vi "Main.vi"() -> ()   [LabVIEW 2016]
doc: "The roboRIO Project template acquires acceleration data from the onboard accelerometer and displays the changes of acceleration values in a waveform chart."
panel:
  out "String":string
  in  "Boolean 1":bool
  in  "Boolean 2":bool
  out "Test 4":bool
  out "Finger 1 (individual) 2":bool
  out "Finger 2 (individual) 2":bool
  out "Finger 3 (individual) 2":bool
  out "Finger 4 (individual)":bool
  out "Finger 5 (individual) 2":bool
  in  "Finger 1 (individual)":bool
  in  "Finger 3 (individual)":bool
  in  "FInger 4 (individual)":bool
  in  "Finger 5 (individual)":bool
  in  "Finger 2 (individual)":bool
  in  "stop":bool
  out "Test 1":bool
  out "Test 2":bool
  out "Test 3":bool
  out "Finger 1 (thumb)":i16(knob) scale=0.0..180.0
  out "Finger 4 (ring)":i16(knob) scale=0.0..180.0
  out "Finger 3 (middle)":i16(knob) scale=0.0..180.0
  out "Finger 2 (index)":i16(knob) scale=0.0..180.0
  out "Finger 5 (little)":i16(knob) scale=0.0..180.0
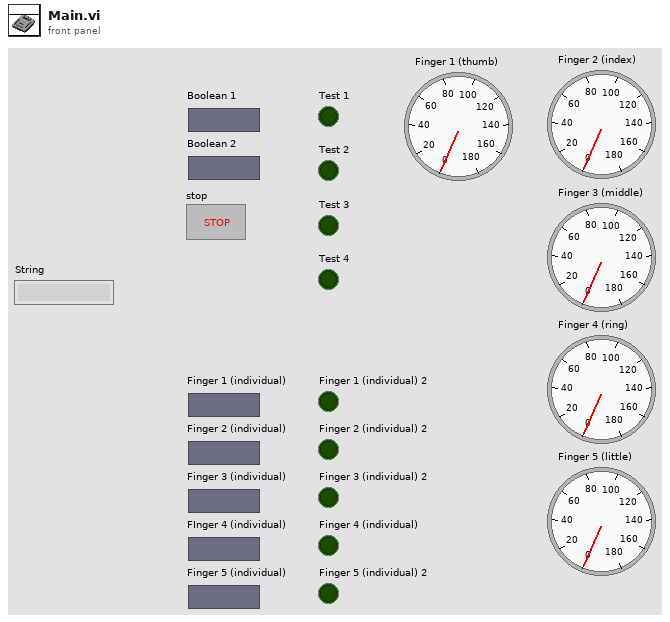
[diagram p1: front panel]
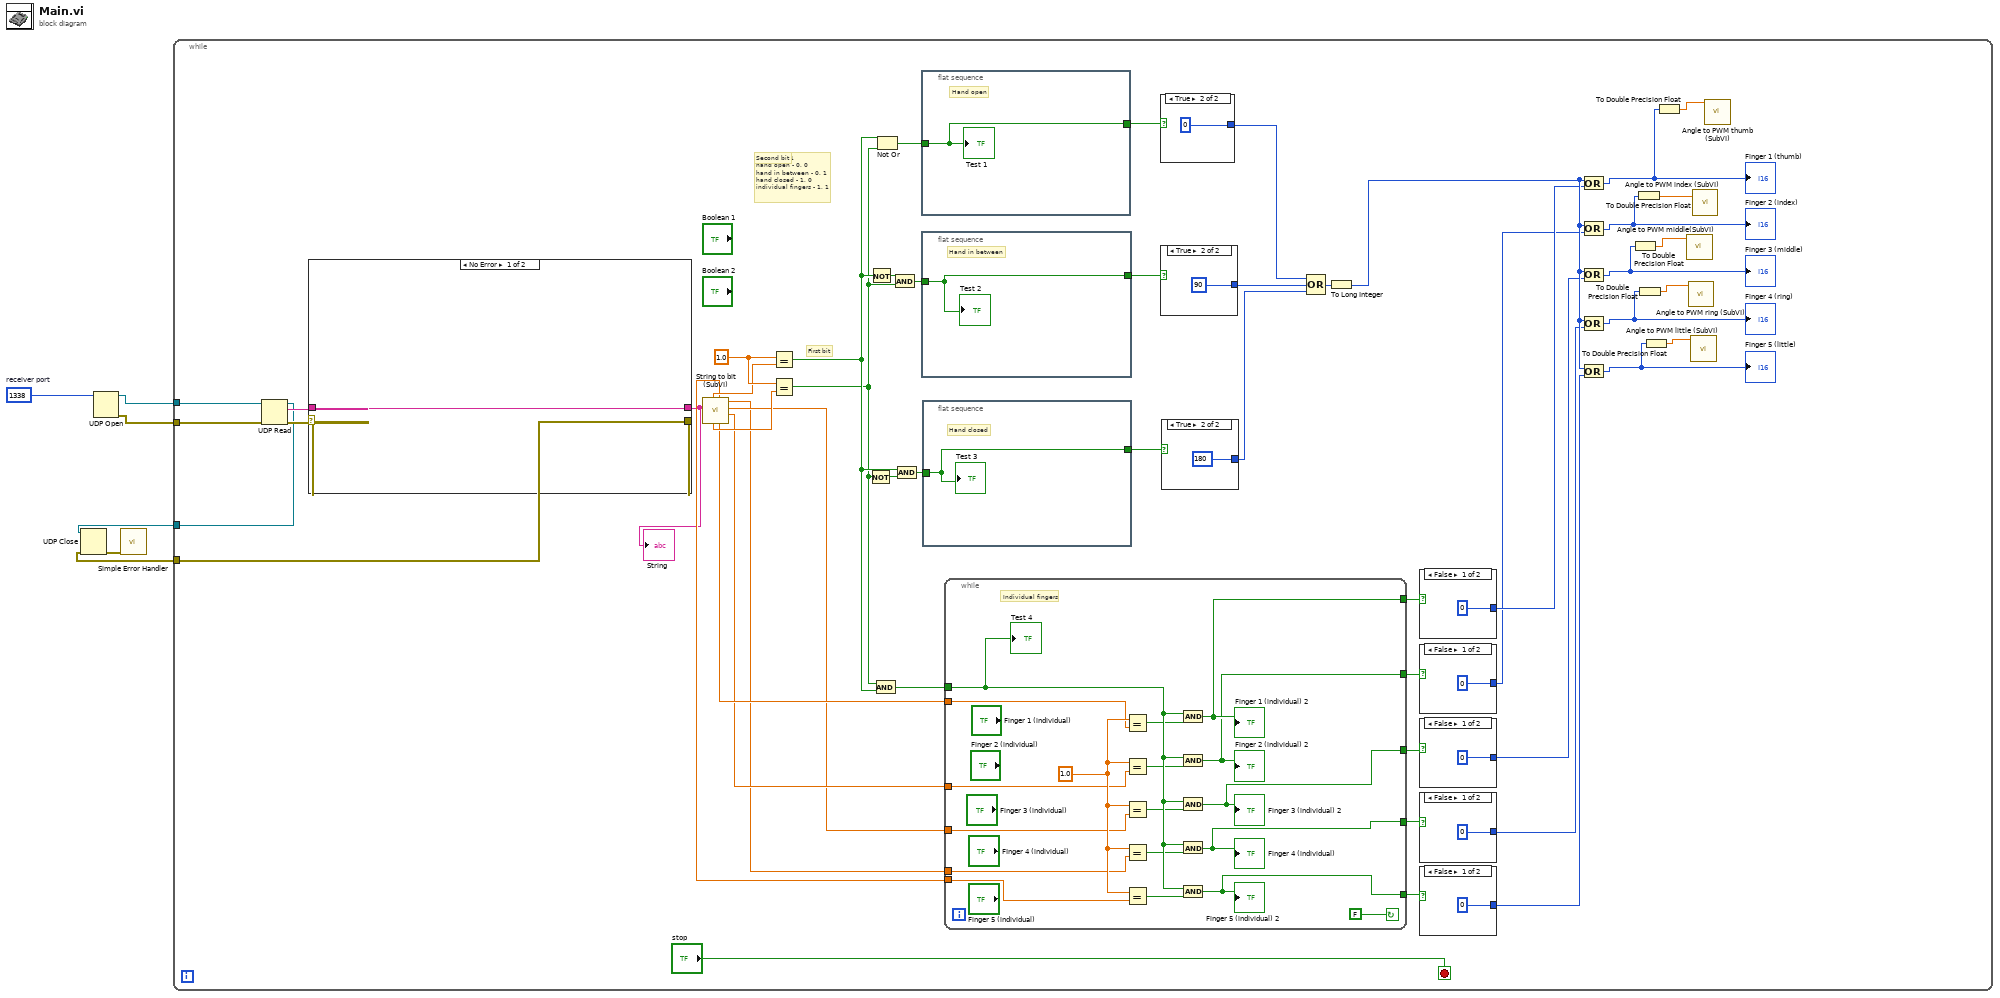
[diagram p0: block diagram]
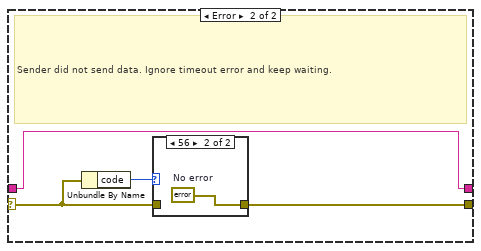
[diagram p2: hidden frame]
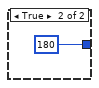
[diagram p4: hidden frame]
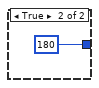
[diagram p5: hidden frame]
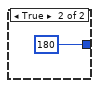
[diagram p6: hidden frame]
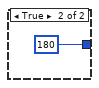
[diagram p7: hidden frame]
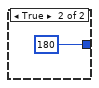
[diagram p8: hidden frame]
diagram:
  w6 = u16 1338  # receiver port
  n1 = UDP Open(11:w6) -> (port=w4:refnum<k16>, 0:w5:errorcluster)  [unwired: 4 in, 1 out]
  n2 = while {
    tunnel: w5 -> [w18]
    tunnel: w4 -> [w17]
    tunnel: [w16] -> w2
    tunnel: [w15] -> w1
    stop <- "stop" stop-if-true
    w38 = 1.0
    # "Second bit"
    # "First bit"
    # "Command 1\nhand open - 0, 0\nhand in between - 0, 1\nhand closed - 1, 0\nindividual fingers - 1, 1"
    n3 = UDP Read(connection ID=w17, 8:w18) -> (data out=w20:string, error out=w19:errorcluster, 3:w16:refnum<k16>)  [unwired: 1 in, 3 out]
    n4 = case shown="No Error" w19 {
      selector: w19 -> [w60 w63]
      tunnel: w20 -> [w59 w61]
      tunnel: [w60 w62] -> w15
      tunnel: [w59 w61] -> w7
      frame No Error {
      }
      frame Error {
        # "Sender did not send data. Ignore timeout error and keep waiting."
        n5 = Unbundle By Name(w63) -> ("code"=w64:i32)
        n6 = case shown="56" w64 {
          tunnel: w63 -> [w65 _]
          tunnel: [w65 w66] -> w62
          frame Default {
          }
          frame 56 {
            w66 = errorcluster {"status"=FALSE, "code"=0, "source"=""}  # No error
          }
        }
      }
    }
    "String" <- w7
    n7 = call "String to bit (SubVI).vi"("String in"=w7) -> ("Pointy finger"=w11:dbl, "Middle finger"=w10:dbl, "Ringfinger"=w9:dbl, "Thumb"=w12:dbl, "Lillfinger"=w8:dbl, "Command LSD"=w14:dbl, "Command MSD"=w13:dbl)  [unwired: 4 in]
    n8 = Equal?(x=w38, y=w13) -> (x = y?=w39:bool)
    n9 = Equal?(x=w38, y=w14) -> (x = y?=w37:bool)
    n10 = Not(x=w37) -> (.not. x?=w57:bool)
    n11 = Not(x=w39) -> (.not. x?=w58:bool)
    n12 = And(x=w37, y=w39) -> (x .and. y?=w56:bool)
    n13 = Not Or(1:w37, 2:w39) -> (0:w55:bool)
    n14 = And(x=w58, y=w37) -> (x .and. y?=w54:bool)
    n15 = And(x=w39, y=w57) -> (x .and. y?=w53:bool)
    n16 = flat-sequence {
      tunnel: w55 -> [w82]
      tunnel: [w82] -> w51
      frame #0 {
        # "Hand open"
        "Test 1" <- w82
      }
    }
    n17 = flat-sequence {
      tunnel: w54 -> [w81]
      tunnel: [w81] -> w52
      frame #0 {
        # "Hand in between"
        "Test 2" <- w81
      }
    }
    n18 = flat-sequence {
      tunnel: w53 -> [w80]
      tunnel: [w80] -> w49
      frame #0 {
        # "Hand closed"
        "Test 3" <- w80
      }
    }
    n19 = while {
      tunnel: w56 -> [w100]
      tunnel: [w98] -> w36
      tunnel: [w97] -> w35
      tunnel: [w96] -> w34
      tunnel: [w95] -> w33
      tunnel: [w94] -> w32
      tunnel: w12 -> [w87]
      tunnel: w11 -> [w86]
      tunnel: w10 -> [w85]
      tunnel: w9 -> [w84]
      tunnel: w8 -> [w83]
      stop <- FALSE continue-if-true
      w93 = 1.0
      # "Individual fingers"
      n20 = Equal?(x=w93, y=w87) -> (x = y?=w92:bool)
      n21 = Equal?(x=w93, y=w86) -> (x = y?=w91:bool)
      n22 = Equal?(x=w93, y=w85) -> (x = y?=w90:bool)
      n23 = Equal?(x=w93, y=w84) -> (x = y?=w89:bool)
      n24 = Equal?(x=w93, y=w83) -> (x = y?=w88:bool)
      n25 = And(x=w100, y=w92) -> (x .and. y?=w98:bool)
      "Finger 1 (individual) 2" <- w98
      n26 = And(x=w100, y=w91) -> (x .and. y?=w97:bool)
      "Finger 2 (individual) 2" <- w97
      n27 = And(x=w100, y=w90) -> (x .and. y?=w96:bool)
      "Finger 3 (individual) 2" <- w96
      n28 = And(x=w100, y=w89) -> (x .and. y?=w95:bool)
      "Finger 4 (individual)" <- w95
      n29 = And(x=w100, y=w88) -> (x .and. y?=w94:bool)
      "Finger 5 (individual) 2" <- w94
      "Test 4" <- w100
    }
    n30 = case shown="True" w51 {
      tunnel: [_ i16 0] -> w50
      frame False {
      }
      frame True {
      }
    }
    n31 = case shown="True" w52 {
      tunnel: [_ i16 90] -> w48
      frame False {
      }
      frame True {
      }
    }
    n32 = case shown="True" w49 {
      tunnel: [_ i16 180] -> w47
      frame False {
      }
      frame True {
      }
    }
    n33 = Compound Arithmetic op=OR(w50, w48, w47) -> (w46:i16)
    n34 = To Long Integer(number=w46) -> (32bit integer=w45:i32)
    n35 = case shown="False" w36 {
      tunnel: [i16 0 i16 180] -> w44
      frame False {
      }
      frame True {
      }
    }
    n36 = case shown="False" w35 {
      tunnel: [i16 0 i16 180] -> w43
      frame False {
      }
      frame True {
      }
    }
    n37 = case shown="False" w34 {
      tunnel: [i16 0 i16 180] -> w42
      frame False {
      }
      frame True {
      }
    }
    n38 = case shown="False" w33 {
      tunnel: [i16 0 i16 180] -> w41
      frame False {
      }
      frame True {
      }
    }
    n39 = case shown="False" w32 {
      tunnel: [i16 0 i16 180] -> w40
      frame False {
      }
      frame True {
      }
    }
    n40 = Compound Arithmetic op=OR(w45, w44) -> (w31:i32)
    "Finger 1 (thumb)" <- w31
    n41 = Compound Arithmetic op=OR(w45, w43) -> (w28:i32)
    "Finger 2 (index)" <- w28
    n42 = Compound Arithmetic op=OR(w45, w42) -> (w27:i32)
    "Finger 3 (middle)" <- w27
    n43 = Compound Arithmetic op=OR(w45, w41) -> (w25:i32)
    "Finger 4 (ring)" <- w25
    n44 = Compound Arithmetic op=OR(w45, w40) -> (w23:i32)
    "Finger 5 (little)" <- w23
    n45 = To Double Precision Float(number=w27) -> (double precision float=w26:dbl)
    n46 = To Double Precision Float(number=w28) -> (double precision float=w29:dbl)
    n47 = To Double Precision Float(number=w25) -> (double precision float=w24:dbl)
    n48 = To Double Precision Float(number=w23) -> (double precision float=w22:dbl)
    n49 = To Double Precision Float(number=w31) -> (double precision float=w30:dbl)
    n50 = call "Angle to PWM middle(SubVI).vi"("Angle in degrees"=w26) -> ()  [unwired: 11 in]
    n51 = call "Angle to PWM ring (SubVI).vi"("Angle in degrees"=w24) -> ()  [unwired: 11 in]
    n52 = call "Angle to PWM little (SubVI).vi"("Angle in degrees"=w22) -> ()  [unwired: 11 in]
    n53 = call "Angle to PWM index (SubVI).vi"("Angle in degrees"=w29) -> ()  [unwired: 11 in]
    n54 = call "Angle to PWM thumb (SubVI).vi"("Angle in degrees"=w30) -> ()  [unwired: 11 in]
  }
  n55 = UDP Close(connection ID=w2, 8:w1) -> (error out=w3:errorcluster)  [unwired: 1 out]
  n56 = call <vilib>:"Simple Error Handler.vi"("error in (no error)"=w3) -> ()  [unwired: 1 in, 8 out]
